vi "GETSTAT.VI"(0 "Function Type":i32(ring)=1, 1 "Context":T1) -> (2 "Context":T1, 3 "Data":u16[](array[numeric]), 4 "Running":bool, 5 "CurCount":i32, 6 "CurIndex":i32, 7 "ErrCode":i32)   [LabVIEW 2009]
doc: "Returns status about background operation currently running."
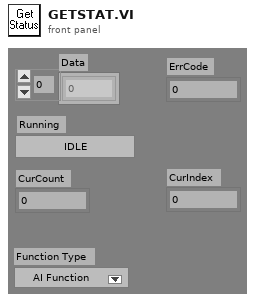
[diagram p1: front panel]
types:
  T1 = cluster{"IntnlBoardNum":i32, "Data":i16[], "Size":i32, "IntnlStatus":i32, "IntnlErrCode":i32, "Alias16":u32, "Reserved":i32}
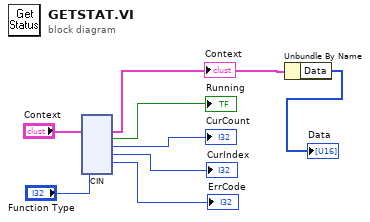
[diagram p0: block diagram]
diagram:
  n1 = cin("Context", "Function Type") -> (w3:T1, →"Running":bool, →"CurCount":i32, →"CurIndex":i32, →"ErrCode":i32)  [unwired: 5 in]
  "Context" <- w3
  n2 = Unbundle By Name(w3) -> ("Data"=→"Data":i16[])
